vi "Setup UI.vi"(8 "error in (no error)":errorcluster, 10 "Set UI to input? (F)":bool, 11 "Varian Magnet Scan in":refnum<class "Varian Magnet Scan.lvclass">) -> (0 "error out":errorcluster, 3 "Varian Magnet Scan out":refnum<class "Varian Magnet Scan.lvclass">)   [LabVIEW 2009, in "Varian Magnet Scan.lvclass"]
doc: "Scanner::Setup is a constructor that has no parameters and faces the user. The Factory calls this VI to let the user configure this Scanner. It is dynamically dispatched in order to let the user choose the type as well as the options of the scanner."
uses:
  Varian Magnet Scan.lvclass
panel:
  in  "Send conds for first point to magnet":bool
  # "Varian Magnet Scan"
  # "PURE VIRTUAL\nMETHOD CALLED!"
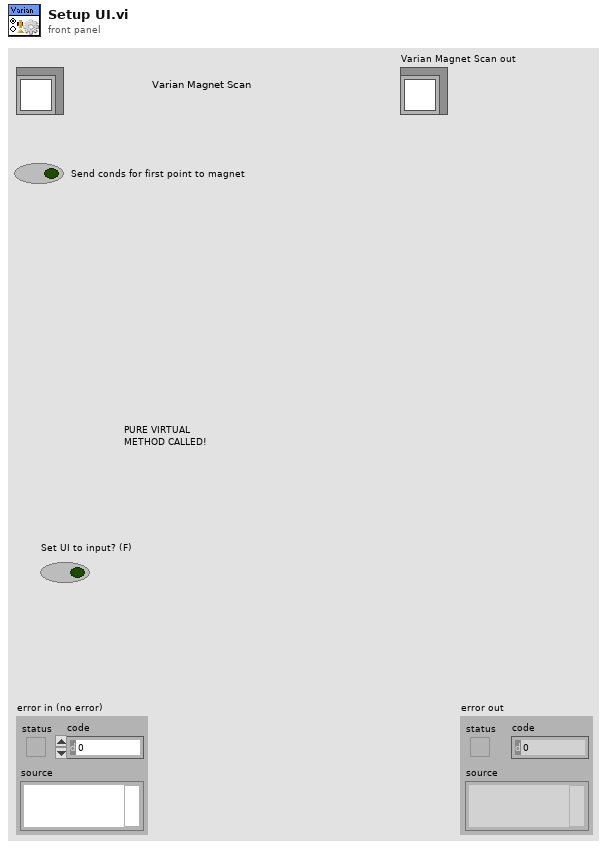
[diagram p1: front panel]
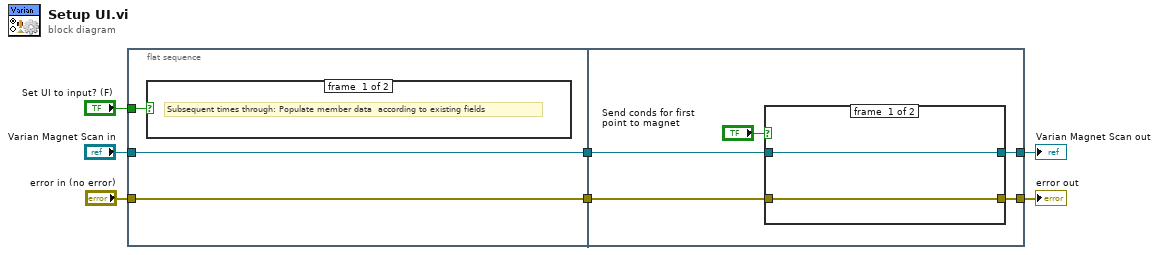
[diagram p0: block diagram]
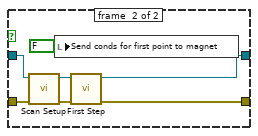
[diagram p3: hidden frame]
diagram:
  n1 = flat-sequence {
    tunnel: "error in (no error)" -> [w9]
    tunnel: "Varian Magnet Scan in" -> [w10]
    tunnel: [w10] -> w5
    tunnel: [w9] -> w4
    tunnel: "Set UI to input? (F)" -> [w8]
    tunnel: [w14] -> w7
    tunnel: [w12] -> w6
    tunnel: w5 -> [w15]
    tunnel: w4 -> [w13]
    frame #0 {
      n2 = case shown="False" w8 {
        frame #0 {
          # "Subsequent times through: Populate member data  according to existing fields"
        }
        frame #1 {
          # "First time through: Populate fields  to existing member data"
        }
      }
    }
    frame #1 {
      n3 = case shown="True" "Send conds for first point to magnet" {
        tunnel: w15 -> [w17 w23]
        tunnel: [w16 w20] -> w12
        tunnel: [w17 w19] -> w14
        tunnel: w13 -> [w16 w18]
        frame #0 {
        }
        frame #1 {
          n4 = call-dynamic "Scan Setup.vi"("error in (no error)"=w18, "Scanner in"=w23) -> ("error out"=w21:errorcluster, "Scanner out"=w22:refnum<class "Varian Magnet Scan.lvclass">)  [unwired: 8 out]
          n5 = local write "Send conds for first point to magnet"(FALSE ("Send conds for first point to PG")) -> ()
          n6 = call-dynamic "First Step.vi"("error in (no error)"=w21, "Varian Magnet Scan.lvclass in"=w22) -> ("error out"=w20:errorcluster, "Varian Magnet Scan.lvclass out"=w19:refnum<class "Varian Magnet Scan.lvclass">)  [unwired: 8 out]
        }
      }
    }
  }
  "error out" <- w6
  "Varian Magnet Scan out" <- w7
